vi "LSMcontroller_v62_updatedpointscan.vi"() -> ()   [LabVIEW 2015] (continued)
                                n918 = Transpose 2D Array(2D array=w3216) -> (transposed array=w3210:u16[][])
                                n919 = Transpose 2D Array(2D array=w3214) -> (transposed array=w3215:sgl[][])
                                n920 = And(x=w3220, y=w3209) -> (x .and. y?=w3222:bool)
                                n921 = local write "img_CH2"(w3215) -> ()
                                n922 = local write "photons/frame"(w3208) -> ()
                                n923 = Array Max & Min(array=w3210) -> (max value=w3211:u16)  [unwired: 3 out]
                                n924 = To Single Precision Float(number=w3210) -> (single precision float=w3213:sgl[][])
                                n925 = case shown="True" w3222 {
                                tunnel: w3221 -> [_ w3226]
                                frame False {
                                }
                                frame True {
                                n926 = Quotient & Remainder(x=w3226, y=u32 2 ("min phot")) -> (floor(x/y)=w3225:u32)  [unwired: 1 out]
                                n927 = Max & Min(x=w3225, y=u32 5) -> (max(x,y)=w3224:u32)  [unwired: 1 out]
                                n928 = local write "min phot"(w3224) -> ()
                                }
                                }
                                n929 = To Double Precision Float(number=w3211) -> (double precision float=w3212:dbl)
                                n930 = local write "img_CH1"(w3213) -> ()
                                n931 = property on="img_CH1" class="IntGraph (strict)"("ZScale.Maximum"=w3212) -> ()  [unwired: 2 in, 2 out]
                                }
                                }
                                }
                                frame #4 {
                                w3230 = u16 1 items=["Stream to disk", "Post process", "real time process"] ("Ring")
                                n932 = local read "T3R Data processing"() -> (w3229:u16)
                                n933 = Equal?(x=w3229, y=w3230) -> (x = y?=w3228:bool)
                                n934 = case shown="False" w3228 {
                                frame False {
                                # "intensity"
                                n935 = local read "Current Average"() -> (w3235:sgl)
                                n936 = local read "image2list"() -> (w3231:u16)
                                n937 = local read "image1list"() -> (w3232:u16)
                                n938 = call "dattoimage.vi"("image2list"=w3231, "Current Average"=w3235, "image1list"=w3232) -> ("image 1 array out"=w3234:sgl[][])  [unwired: 1 out]
                                n939 = Transpose 2D Array(2D array=w3234) -> (transposed array=w3233:sgl[][])
                                n940 = local write "img_CH2"(w3233) -> ()
                                }
                                frame True {
                                }
                                }
                                }
                                }
                              }
                              frame Enabled {
                              }
                            }
                          }
                        }
                        n941 = local write "64bit disabled"(TRUE ("64bit disabled")) -> ()
                      }
                      frame #9 {
                        n942 = call "2pparameters.vi"("command"="get") -> ("params out"=w3238:T10)  [unwired: 1 in]
                        n943 = Unbundle By Name(w3238) -> ("auto OD"=w3237:bool)
                        n944 = case shown="True" w3237 {
                          frame False {
                          }
                          frame True {
                            n945 = call "configuration.vi"("command"="get") -> ("config out"=w3241:T11)  [unwired: 2 in, 1 out]
                            n946 = call "2pparameters.vi"("command"="get") -> ("params out"=w3244:T10)  [unwired: 1 in]
                            n947 = Unbundle By Name(w3241) -> ("image OD"=w3239:u16)
                            n948 = Unbundle By Name(w3244) -> ("ODfilt"=w3240:u16)
                            n949 = call "filterwheelcontrol_nothorlabslib.vi"("Current OD filt"=w3239, "New ODfilt"=w3240) -> ()  [unwired: 1 in]
                          }
                        }
                        n950 = call "reset AO_DO_v3.vi"() -> ()  [unwired: 12 in]
                      }
                      frame #10 {
                        n951 = stacked-sequence {
                          tunnel: w3258 -> [w3261 _ _ _ _ _]
                          tunnel: w3257 -> [w3260 _ _ _ _ _]
                          tunnel: w3256 -> [w3259 _ _ _ _ _]
                          tunnel: w3255 -> [_ w3310 _ _ _ _]
                          tunnel: w3254 -> [_ w3309 w3364 w3461 _ _]
                          tunnel: w3253 -> [_ w3308 w3363 w3460 _ _]
                          tunnel: w3252 -> [_ _ w3362 _ _ _]
                          tunnel: w3251 -> [_ _ w3361 _ _ _]
                          tunnel: w3250 -> [_ _ _ w3459 _ _]
                          tunnel: w3249 -> [_ _ _ w3458 _ _]
                          tunnel: w3248 -> [_ _ w3359 _ _ _]
                          tunnel: w3247 -> [_ _ w3358 _ _ _]
                          tunnel: w3246 -> [_ _ _ w3456 _ _]
                          tunnel: w3245 -> [_ _ _ w3455 _ _]
                          frame #0 {
                            n952 = case shown="False" w3261 {
                              tunnel: w3260 -> [_ w3283]
                              tunnel: w3259 -> [_ w3282]
                              frame True {
                                n953 = stacked-sequence {
                                seq-local: [w3262 _ _] -> [_ w3274 w3279]
                                frame #0 {
                                n954 = call "configuration.vi"("command"="get") -> ("config out"=w3268:T11)  [unwired: 2 in, 1 out]
                                n955 = Unbundle By Name(w3268) -> ("Voltage to Xgalvo"=w3265:i32)
                                n956 = call "2pparameters.vi"("command"="get") -> ("params out"=w3266:T10)  [unwired: 1 in]
                                n957 = in-place {
                                in-place-border: w3265 -> [w3273]
                                in-place-border: [w3270] -> w3262
                                n958 = in-place-cluster #9(w3266) -> ("aAO"=w3272:u32[])
                                n959 = call "remove channel from active arrayv2.vi"("line array in"=w3272, "line to remove"=w3273) -> ("line array out"=w3271:u32[], "index"=w3270:i32)  [unwired: 1 out]
                                n960 = in-place-cluster #9("aAO"=w3271) -> (w3263:T10)
                                }
                                n961 = call "2pparameters.vi"("Params in"=w3263, "command"="set") -> ()  [unwired: 1 out]
                                }
                                frame #1 {
                                n962 = call "waveformparamsv2.vi"("command"="rem AO", "index"=w3274) -> ()  [unwired: 3 in, 3 out]
                                }
                                frame #2 {
                                n963 = call "waveformsAObuffer.vi"("command"="get") -> ("AO wf out"=w3280:waveform(dbl)[])  [unwired: 1 in]
                                n964 = Delete From Array(array=w3280, length=1, index=w3279) -> (array with subset deleted=w3276:waveform(dbl)[])  [unwired: 1 out]
                                n965 = call "waveformsAObuffer.vi"("AO wf in"=w3276, "command"="set") -> ()  [unwired: 1 out]
                                }
                                }
                              }
                              frame False {
                                n966 = stacked-sequence {
                                seq-local: [w3284 _ _] -> [_ w3292 w3303]
                                tunnel: w3283 -> [_ w3291 _]
                                tunnel: w3282 -> [_ _ w3302]
                                frame #0 {
                                n967 = call "configuration.vi"("command"="get") -> ("config out"=w3289:T11)  [unwired: 2 in, 1 out]
                                n968 = Unbundle By Name(w3289) -> ("Voltage to Xgalvo"=w3285:i32)
                                n969 = call "2pparameters.vi"("command"="get") -> ("params out"=w3288:T10)  [unwired: 1 in]
                                n970 = Unbundle By Name(w3288) -> ("aAO"=w3286:u32[])
                                n971 = Search 1D Array(1D array=w3286, element=w3285) -> (index of element=w3284:i32)  [unwired: 1 in]
                                }
                                frame #1 {
                                n972 = call "waveformparamsv2.vi"("command"="get") -> ("Params out"=w3295:T14)  [unwired: 4 in, 2 out]
                                n973 = in-place {
                                in-place-border: w3292 -> [w3299]
                                in-place-border: w3291 -> [w3298]
                                n974 = in-place-cluster #10(w3295) -> ("AO parameters"=w3300:T15)
                                n975 = in-place {
                                in-place-border: w3298 -> [w3301]
                                n976 = in-place-array #11(w3300, w3299) -> ()  [unwired: 1 out]
                                n977 = in-place-array #11(w3301) -> (w3297:T15)  [unwired: 1 out]
                                }
                                n978 = in-place-cluster #10("AO parameters"=w3297) -> (w3293:T14)
                                }
                                n979 = call "waveformparamsv2.vi"("command"="set", "Params in"=w3293) -> ()  [unwired: 3 in, 3 out]
                                }
                                frame #2 {
                                n980 = call "waveformsAObuffer.vi"("command"="get") -> ("AO wf out"=w3306:waveform(dbl)[])  [unwired: 1 in]
                                n981 = Replace Array Subset(array=w3306, new element=w3302, index=w3303) -> (w3304:waveform(dbl)[])
                                n982 = call "waveformsAObuffer.vi"("AO wf in"=w3304, "command"="set") -> ()  [unwired: 1 out]
                                }
                                }
                              }
                            }
                          }
                          frame #1 {
                            n983 = case shown="True" w3310 {
                              tunnel: w3309 -> [_ w3332]
                              tunnel: w3308 -> [_ w3331]
                              frame True {
                                n984 = stacked-sequence {
                                seq-local: [w3311 _ _] -> [_ w3323 w3328]
                                frame #0 {
                                n985 = call "configuration.vi"("command"="get") -> ("config out"=w3317:T11)  [unwired: 2 in, 1 out]
                                n986 = Unbundle By Name(w3317) -> ("Voltage to Ygalvo"=w3314:i32)
                                n987 = call "2pparameters.vi"("command"="get") -> ("params out"=w3315:T10)  [unwired: 1 in]
                                n988 = in-place {
                                in-place-border: w3314 -> [w3322]
                                in-place-border: [w3319] -> w3311
                                n989 = in-place-cluster #12(w3315) -> ("aAO"=w3321:u32[])
                                n990 = call "remove channel from active arrayv2.vi"("line array in"=w3321, "line to remove"=w3322) -> ("line array out"=w3320:u32[], "index"=w3319:i32)  [unwired: 1 out]
                                n991 = in-place-cluster #12("aAO"=w3320) -> (w3312:T10)
                                }
                                n992 = call "2pparameters.vi"("Params in"=w3312, "command"="set") -> ()  [unwired: 1 out]
                                }
                                frame #1 {
                                n993 = call "waveformparamsv2.vi"("command"="rem AO", "index"=w3323) -> ()  [unwired: 3 in, 3 out]
                                }
                                frame #2 {
                                n994 = call "waveformsAObuffer.vi"("command"="get") -> ("AO wf out"=w3329:waveform(dbl)[])  [unwired: 1 in]
                                n995 = Delete From Array(array=w3329, length=1, index=w3328) -> (array with subset deleted=w3325:waveform(dbl)[])  [unwired: 1 out]
                                n996 = call "waveformsAObuffer.vi"("AO wf in"=w3325, "command"="set") -> ()  [unwired: 1 out]
                                }
                                }
                              }
                              frame False {
                                n997 = stacked-sequence {
                                seq-local: [w3333 _ _] -> [_ w3341 w3352]
                                tunnel: w3332 -> [_ w3340 _]
                                tunnel: w3331 -> [_ _ w3351]
                                frame #0 {
                                n998 = call "configuration.vi"("command"="get") -> ("config out"=w3338:T11)  [unwired: 2 in, 1 out]
                                n999 = Unbundle By Name(w3338) -> ("Voltage to Ygalvo"=w3334:i32)
                                n1000 = call "2pparameters.vi"("command"="get") -> ("params out"=w3337:T10)  [unwired: 1 in]
                                n1001 = Unbundle By Name(w3337) -> ("aAO"=w3335:u32[])
                                n1002 = Search 1D Array(1D array=w3335, element=w3334) -> (index of element=w3333:i32)  [unwired: 1 in]
                                }
                                frame #1 {
                                n1003 = call "waveformparamsv2.vi"("command"="get") -> ("Params out"=w3344:T14)  [unwired: 4 in, 2 out]
                                n1004 = in-place {
                                in-place-border: w3341 -> [w3348]
                                in-place-border: w3340 -> [w3347]
                                n1005 = in-place-cluster #13(w3344) -> ("AO parameters"=w3349:T15)
                                n1006 = in-place {
                                in-place-border: w3347 -> [w3350]
                                n1007 = in-place-array #14(w3349, w3348) -> ()  [unwired: 1 out]
                                n1008 = in-place-array #14(w3350) -> (w3346:T15)  [unwired: 1 out]
                                }
                                n1009 = in-place-cluster #13("AO parameters"=w3346) -> (w3342:T14)
                                }
                                n1010 = call "waveformparamsv2.vi"("command"="set", "Params in"=w3342) -> ()  [unwired: 3 in, 3 out]
                                }
                                frame #2 {
                                n1011 = call "waveformsAObuffer.vi"("command"="get") -> ("AO wf out"=w3355:waveform(dbl)[])  [unwired: 1 in]
                                n1012 = Replace Array Subset(array=w3355, new element=w3351, index=w3352) -> (w3353:waveform(dbl)[])
                                n1013 = call "waveformsAObuffer.vi"("AO wf in"=w3353, "command"="set") -> ()  [unwired: 1 out]
                                }
                                }
                              }
                            }
                          }
                          frame #2 {
                            n1014 = Build Array(w3359, w3358) -> (w3357:bool[])
                            n1015 = Boolean Array To Number(Boolean array=w3357) -> (number=w3360:u32)
                            n1016 = case shown="0" w3360 {
                              tunnel: w3364 -> [_ _ w3407]
                              tunnel: w3363 -> [_ _ w3406]
                              tunnel: w3362 -> [_ w3386 w3404]
                              tunnel: w3361 -> [_ w3385 w3405]
                              frame 1, Default {
                                n1017 = stacked-sequence {
                                seq-local: [w3365 _ _] -> [_ w3377 w3382]
                                frame #0 {
                                n1018 = call "configuration.vi"("command"="get") -> ("config out"=w3371:T11)  [unwired: 2 in, 1 out]
                                n1019 = Unbundle By Name(w3371) -> ("2P shutter"=w3368:i32)
                                n1020 = call "2pparameters.vi"("command"="get") -> ("params out"=w3369:T10)  [unwired: 1 in]
                                n1021 = in-place {
                                in-place-border: w3368 -> [w3376]
                                in-place-border: [w3373] -> w3365
                                n1022 = in-place-cluster #15(w3369) -> ("aDO"=w3375:u32[])
                                n1023 = call "remove channel from active arrayv2.vi"("line array in"=w3375, "line to remove"=w3376) -> ("line array out"=w3374:u32[], "index"=w3373:i32)  [unwired: 1 out]
                                n1024 = in-place-cluster #15("aDO"=w3374) -> (w3366:T10)
                                }
                                n1025 = call "2pparameters.vi"("Params in"=w3366, "command"="set") -> ()  [unwired: 1 out]
                                }
                                frame #1 {
                                n1026 = call "waveformparamsv2.vi"("command"="rem DO", "index"=w3377) -> ()  [unwired: 3 in, 3 out]
                                }
                                frame #2 {
                                n1027 = call "waveformsDObuffer.vi"("command"="get") -> ("DO wf out"=w3383:digitalwaveform[])  [unwired: 1 in]
                                n1028 = Delete From Array(array=w3383, length=1, index=w3382) -> (array with subset deleted=w3379:digitalwaveform[])  [unwired: 1 out]
                                n1029 = call "waveformsDObuffer.vi"("DO wf in"=w3379, "command"="set") -> ()  [unwired: 1 out]
                                }
                                }
                              }
                              frame 2 {
                                n1030 = stacked-sequence {
                                tunnel: w3386 -> [_ w3397 _]
                                tunnel: w3385 -> [_ _ w3401]
                                frame #0 {
                                n1031 = call "configuration.vi"("command"="get") -> ("config out"=w3388:T11)  [unwired: 2 in, 1 out]
                                n1032 = call "2pparameters.vi"("command"="get") -> ("params out"=w3392:T10)  [unwired: 1 in]
                                n1033 = Unbundle By Name(w3388) -> ("2P shutter"=w3387:i32)
                                n1034 = in-place {
                                in-place-border: w3387 -> [w3396]
                                n1035 = in-place-cluster #16(w3392) -> ("aDO"=w3395:u32[])
                                n1036 = call "add channel to active arrayv2.vi"("line array in"=w3395, "line to add"=w3396) -> ("line array out"=w3394:u32[])  [unwired: 2 out]
                                n1037 = in-place-cluster #16("aDO"=w3394) -> (w3390:T10)
                                }
                                n1038 = call "2pparameters.vi"("Params in"=w3390, "command"="set") -> ()  [unwired: 1 out]
                                }
                                frame #1 {
                                n1039 = call "waveformparamsv2.vi"("command"="add DO", "add DO"=w3397) -> ()  [unwired: 3 in, 3 out]
                                }
                                frame #2 {
                                n1040 = call "waveformsDObuffer.vi"("command"="get") -> ("DO wf out"=w3402:digitalwaveform[])  [unwired: 1 in]
                                n1041 = Build Array (concatenate)(w3402, w3401) -> (w3400:digitalwaveform[])
                                n1042 = call "waveformsDObuffer.vi"("DO wf in"=w3400, "command"="set") -> ()  [unwired: 1 out]
                                }
                                }
                              }
                              frame 0 {
                                n1043 = stacked-sequence {
                                seq-local: [w3408 _ _] -> [_ w3416 w3438]
                                tunnel: w3407 -> [_ _ _]
                                tunnel: w3406 -> [_ _ _]
                                tunnel: w3405 -> [_ _ w3437]
                                tunnel: w3404 -> [_ w3415 _]
                                frame #0 {
                                n1044 = call "configuration.vi"("command"="get") -> ("config out"=w3413:T11)  [unwired: 2 in, 1 out]
                                n1045 = call "2pparameters.vi"("command"="get") -> ("params out"=w3412:T10)  [unwired: 1 in]
                                n1046 = Unbundle By Name(w3413) -> ("2P shutter"=w3409:i32)
                                n1047 = Unbundle By Name(w3412) -> ("aDO"=w3410:u32[])
                                n1048 = Search 1D Array(1D array=w3410, element=w3409) -> (index of element=w3408:i32)  [unwired: 1 in]
                                }
                                frame #1 {
                                n1049 = call "2pparameters.vi"("command"="get") -> ("params out"=w3419:T10)  [unwired: 1 in]
                                n1050 = Unbundle By Name(w3419) -> ("wavdet"=w3417:bool, "autoshutter"=w3418:bool)
                                n1051 = case shown="True" w3418 {
                                tunnel: w3416 -> [_ w3423]
                                tunnel: w3417 -> [_ w3422]
                                tunnel: w3415 -> [_ w3421]
                                frame False {
                                }
                                frame True {
                                n1052 = case shown="False" w3422 {
                                tunnel: w3423 -> [w3427 _]
                                tunnel: w3421 -> [w3425 _]
                                frame False {
                                n1053 = Index Array(array=w3425, index=0) -> (element=w3424:T18)
                                n1054 = call "waveformparamsv2.vi"("command"="get") -> ("Params out"=w3430:T14)  [unwired: 4 in, 2 out]
                                n1055 = in-place {
                                in-place-border: w3427 -> [w3434]
                                in-place-border: w3424 -> [w3432]
                                n1056 = in-place-cluster #17(w3430) -> ("DO parameters"=w3435:T17)
                                n1057 = in-place {
                                in-place-border: w3432 -> [w3436]
                                n1058 = in-place-array #18(w3435, w3434) -> ()  [unwired: 1 out]
                                n1059 = in-place-array #18(w3436) -> (w3433:T17)  [unwired: 1 out]
                                }
                                n1060 = in-place-cluster #17("DO parameters"=w3433) -> (w3428:T14)
                                }
                                n1061 = call "waveformparamsv2.vi"("command"="set", "Params in"=w3428) -> ()  [unwired: 3 in, 3 out]
                                }
                                frame True {
                                }
                                }
                                }
                                }
                                }
                                frame #2 {
                                n1062 = call "2pparameters.vi"("command"="get") -> ("params out"=w3441:T10)  [unwired: 1 in]
                                n1063 = Unbundle By Name(w3441) -> ("wavdet"=w3439:bool, "autoshutter"=w3440:bool)
                                n1064 = case shown="True" w3440 {
                                tunnel: w3438 -> [_ w3445]
                                tunnel: w3439 -> [_ w3444]
                                tunnel: w3437 -> [_ w3443]
                                frame False {
                                }
                                frame True {
                                n1065 = case shown="False" w3444 {
                                tunnel: w3445 -> [w3449 _]
                                tunnel: w3443 -> [w3448 _]
                                frame False {
                                n1066 = Index Array(array=w3448, index=0) -> (element=w3446:digitalwaveform)
                                n1067 = call "waveformsDObuffer.vi"("command"="get") -> ("DO wf out"=w3451:digitalwaveform[])  [unwired: 1 in]
                                n1068 = Replace Array Subset(array=w3451, new element=w3446, index=w3449) -> (w3453:digitalwaveform[])
                                n1069 = call "waveformsDObuffer.vi"("DO wf in"=w3453, "command"="set") -> ()  [unwired: 1 out]
                                }
                                frame True {
                                }
                                }
                                }
                                }
                                }
                                }
                              }
                            }
                          }
                          frame #3 {
                            n1070 = Build Array(w3456, w3455) -> (w3457:bool[])
                            n1071 = Boolean Array To Number(Boolean array=w3457) -> (number=w3454:u32)
                            n1072 = case shown="0" w3454 {
                              tunnel: w3461 -> [_ _ w3504]
                              tunnel: w3460 -> [_ _ w3503]
                              tunnel: w3459 -> [_ w3483 w3501]
                              tunnel: w3458 -> [_ w3482 w3502]
                              frame 1, Default {
                                n1073 = stacked-sequence {
                                seq-local: [w3462 _ _] -> [_ w3474 w3479]
                                frame #0 {
                                n1074 = call "configuration.vi"("command"="get") -> ("config out"=w3468:T11)  [unwired: 2 in, 1 out]
                                n1075 = Unbundle By Name(w3468) -> ("LT timestamp"=w3465:u32)
                                n1076 = call "2pparameters.vi"("command"="get") -> ("params out"=w3466:T10)  [unwired: 1 in]
                                n1077 = in-place {
                                in-place-border: w3465 -> [w3473]
                                in-place-border: [w3470] -> w3462
                                n1078 = in-place-cluster #19(w3466) -> ("aDO"=w3472:u32[])
                                n1079 = call "remove channel from active arrayv2.vi"("line array in"=w3472, "line to remove"=w3473) -> ("line array out"=w3471:u32[], "index"=w3470:i32)  [unwired: 1 out]
                                n1080 = in-place-cluster #19("aDO"=w3471) -> (w3463:T10)
                                }
                                n1081 = call "2pparameters.vi"("Params in"=w3463, "command"="set") -> ()  [unwired: 1 out]
                                }
                                frame #1 {
                                n1082 = call "waveformparamsv2.vi"("command"="rem DO", "index"=w3474) -> ()  [unwired: 3 in, 3 out]
                                }
                                frame #2 {
                                n1083 = call "waveformsDObuffer.vi"("command"="get") -> ("DO wf out"=w3480:digitalwaveform[])  [unwired: 1 in]
                                n1084 = Delete From Array(array=w3480, length=1, index=w3479) -> (array with subset deleted=w3476:digitalwaveform[])  [unwired: 1 out]
                                n1085 = call "waveformsDObuffer.vi"("DO wf in"=w3476, "command"="set") -> ()  [unwired: 1 out]
                                }
                                }
                              }
                              frame 2 {
                                n1086 = stacked-sequence {
                                tunnel: w3483 -> [_ _ w3496]
                                tunnel: w3482 -> [_ w3494 _]
                                frame #0 {
                                n1087 = call "configuration.vi"("command"="get") -> ("config out"=w3485:T11)  [unwired: 2 in, 1 out]
                                n1088 = Unbundle By Name(w3485) -> ("LT timestamp"=w3484:u32)
                                n1089 = call "2pparameters.vi"("command"="get") -> ("params out"=w3489:T10)  [unwired: 1 in]
                                n1090 = in-place {
                                in-place-border: w3484 -> [w3493]
                                n1091 = in-place-cluster #20(w3489) -> ("aDO"=w3492:u32[])
                                n1092 = call "add channel to active arrayv2.vi"("line array in"=w3492, "line to add"=w3493) -> ("line array out"=w3491:u32[])  [unwired: 2 out]
                                n1093 = in-place-cluster #20("aDO"=w3491) -> (w3487:T10)
                                }
                                n1094 = call "2pparameters.vi"("Params in"=w3487, "command"="set") -> ()  [unwired: 1 out]
                                }
                                frame #1 {
                                n1095 = call "waveformparamsv2.vi"("command"="add DO", "add DO"=w3494) -> ()  [unwired: 3 in, 3 out]
                                }
                                frame #2 {
                                n1096 = call "waveformsDObuffer.vi"("command"="get") -> ("DO wf out"=w3499:digitalwaveform[])  [unwired: 1 in]
                                n1097 = Build Array (concatenate)(w3499, w3496) -> (w3498:digitalwaveform[])
                                n1098 = call "waveformsDObuffer.vi"("DO wf in"=w3498, "command"="set") -> ()  [unwired: 1 out]
                                }
                                }
                              }
                              frame 0 {
                                n1099 = stacked-sequence {
                                seq-local: [w3505 _ _] -> [_ w3515 w3532]
                                tunnel: w3504 -> [_ _ _]
                                tunnel: w3503 -> [_ _ _]
                                tunnel: w3502 -> [_ w3512 _]
                                tunnel: w3501 -> [_ _ w3531]
                                frame #0 {
                                n1100 = call "configuration.vi"("command"="get") -> ("config out"=w3510:T11)  [unwired: 2 in, 1 out]
                                n1101 = Unbundle By Name(w3510) -> ("LT timestamp"=w3506:u32)
                                n1102 = call "2pparameters.vi"("command"="get") -> ("params out"=w3509:T10)  [unwired: 1 in]
                                n1103 = Unbundle By Name(w3509) -> ("aDO"=w3507:u32[])
                                n1104 = Search 1D Array(1D array=w3507, element=w3506) -> (index of element=w3505:i32)  [unwired: 1 in]
                                }
                                frame #1 {
                                n1105 = local read "Measurement"() -> (w3514:T4)
                                n1106 = To Unsigned Long Integer(number=w3514) -> (unsigned 32bit integer=w3513:u32)
                                n1107 = case shown="5..7" w3513 {
                                tunnel: w3515 -> [_ w3519]
                                tunnel: w3512 -> [_ w3516]
                                frame 0..4, Default {
                                }
                                frame 5..7 {
                                n1108 = Index Array(array=w3516, index=0) -> (element=w3517:T18)
                                n1109 = call "waveformparamsv2.vi"("command"="get") -> ("Params out"=w3522:T14)  [unwired: 4 in, 2 out]
                                n1110 = in-place {
                                in-place-border: w3519 -> [w3526]
                                in-place-border: w3517 -> [w3524]
                                n1111 = in-place-cluster #21(w3522) -> ("DO parameters"=w3527:T17)
                                n1112 = in-place {
                                in-place-border: w3524 -> [w3528]
                                n1113 = in-place-array #22(w3527, w3526) -> ()  [unwired: 1 out]
                                n1114 = in-place-array #22(w3528) -> (w3525:T17)  [unwired: 1 out]
                                }
                                n1115 = in-place-cluster #21("DO parameters"=w3525) -> (w3520:T14)
                                }
                                n1116 = call "waveformparamsv2.vi"("command"="set", "Params in"=w3520) -> ()  [unwired: 3 in, 3 out]
                                }
                                }
                                }
                                frame #2 {
                                n1117 = local read "Measurement"() -> (w3530:T4)
                                n1118 = To Unsigned Long Integer(number=w3530) -> (unsigned 32bit integer=w3529:u32)
                                n1119 = case shown="5..7" w3529 {
                                tunnel: w3532 -> [_ w3536]
                                tunnel: w3531 -> [_ w3534]
                                frame 0..4, Default {
                                }
                                frame 5..7 {
                                n1120 = Index Array(array=w3534, index=0) -> (element=w3533:digitalwaveform)
                                n1121 = call "waveformsDObuffer.vi"("command"="get") -> ("DO wf out"=w3538:digitalwaveform[])  [unwired: 1 in]
                                n1122 = Replace Array Subset(array=w3538, new element=w3533, index=w3536) -> (w3540:digitalwaveform[])
                                n1123 = call "waveformsDObuffer.vi"("DO wf in"=w3540, "command"="set") -> ()  [unwired: 1 out]
                                }
                                }
                                }
                                }
                              }
                            }
                          }
                          frame #4 {
                            n1124 = call "Used AO lines.vi"() -> ("used AO names"=w3543:string[], "used AO lines"=w3541:tag[])  [unwired: 2 in]
                            n1125 = control-ref of="Analog Lines Plot"() -> (w3542:refnum<vi>)
                            n1126 = control-ref of="Digital Lines Plot"() -> (w3544:refnum<vi>)
                            n1127 = call "Used DO lines.vi"() -> ("used DO names"=w3545:string[], "used DO lines"=w3546:tag[])  [unwired: 2 in]
                            n1128 = local write "Analog Used Lines"(w3541) -> ()
                            n1129 = local write "Analog Used Names"(w3543) -> ()
                            n1130 = local write "Digital Used Lines"(w3546) -> ()
                            n1131 = local write "Digital Used Names"(w3545) -> ()
                            n1132 = call "prepDOWaveplot.vi"("DigitalGraph in"=w3544, "used DO names"=w3545) -> ()  [unwired: 1 in]
                            n1133 = call "prepAOWaveplot.vi"("WaveformGraph in"=w3542, "Analog Used Names"=w3543) -> ()  [unwired: 1 in]
                          }
                          frame #5 {
                            n1134 = local read "Meastab"() -> (w3561:enum32{"X-Y Image", "Linescan", "Timetrace"})
                            n1135 = property on="refwf" class="Ring (strict)"() -> ("RingText.Text"=w3558:string)  [unwired: 2 in, 2 out]
                            n1136 = case shown="\"Timetrace\"" w3561 {
                              tunnel: [w3563 w3564] -> w3562
                              frame "X-Y Image", Default {
                                n1137 = local read "Sampling rate"() -> (w3563:dbl)
                              }
                              frame "Timetrace" {
                                n1138 = local read "srateAODOtt"() -> (w3564:dbl)
                              }
                            }
                            n1139 = call "waveformsAObuffer.vi"("command"="get") -> ("AO wf out"=w3549:waveform(dbl)[])  [unwired: 1 in]
                            n1140 = local read "wavdet"() -> (w3559:bool)
                            n1141 = call "waveformsDObuffer.vi"("command"="get") -> ("DO wf out"=w3553:digitalwaveform[])  [unwired: 1 in]
                            n1142 = call "correctwaveformsizetemp.vi"("new sampling frequency (Hz)"=w3562, "start"=FALSE, "reference waveforms to"=w3558, "Analog waveforms in"=w3549, "stop"=TRUE, "Digital waveforms in"=w3553) -> ("analog wf out"=w3555:waveform(dbl)[], "Digital wf out"=w3557:digitalwaveform[], "measpoints"=w3560:i32)
                            n1143 = local write "Analog Lines Plot"(w3555) -> ()
                            n1144 = call "GetNumCamFramesv2.vi"("Digital Waveform Graph"=w3557) -> ("Numeric"=w3556:i32)  [unwired: 10 in]
                            n1145 = local write "Digital Lines Plot"(w3557) -> ()
                            n1146 = call "waveformsDObuffer.vi"("DO wf in"=w3557, "command"="set") -> ()  [unwired: 1 out]
                            n1147 = call "waveformsAObuffer.vi"("AO wf in"=w3555, "command"="set") -> ()  [unwired: 1 out]
                            n1148 = local write "Total Camera Frames"(w3556) -> ()
                            n1149 = case shown="True" w3559 {
                              tunnel: w3560 -> [_ w3565]
                              frame False {
                              }
                              frame True {
                                n1150 = local write "# of frames"(w3565) -> ()
                              }
                            }
                          }
                        }
                        n1151 = call "stoperaseCI.vi"() -> ()  [unwired: 12 in]
                        n1152 = call "stoperaseDO_img.vi"() -> ()  [unwired: 12 in]
                        n1153 = call "stoperaseAO_img.vi"() -> ()  [unwired: 12 in]
                        n1154 = call "stoperaseAI_img.vi"() -> ()  [unwired: 12 in]
                      }
                      frame #11 {
                        w3573 = FALSE ("Value (Signaling)")
                        n1155 = local read "save\ndata"() -> (w3566:bool)
                        n1156 = local read "save\ndata"() -> (w3567:bool)
                        n1157 = property on="Stop" class="Bool (strict)"("Visible"=FALSE, "DisabledEnum"=T7."Disabled" ("Disabled")) -> ()  [unwired: 2 in, 2 out]
                        n1158 = case shown="True" w3566 {
                          frame False {
                          }
                          frame True {
                            n1159 = call "closetiffs.vi"() -> ()  [unwired: 12 in]
                          }
                        }
                        n1160 = case shown="True" w3567 {
                          tunnel: w3568 -> [_ w3574]
                          frame False {
                          }
                          frame True {
                            n1161 = local read "filename prefix"() -> (w3576:string)
                            n1162 = local read "data dir"() -> (w3575:path)
                            n1163 = call "savetimestamps.vi"("timestamp"=w3574, "filename prefix in"=w3576, "data dir in"=w3575) -> ()  [unwired: 1 in]
                            n1164 = call "saveparams.vi"("filename prefix in"=w3576, "data dir in"=w3575) -> ()  [unwired: 2 in]
                          }
                        }
                        n1165 = property on="Start" class="Bool (strict)"("Visible"=TRUE, "DisabledEnum"=T7."Enabled" ("Disabled")) -> ()  [unwired: 2 in, 2 out]
                        n1166 = property on="Start" class="Bool (strict)"("Val(Sgnl)"=w3573) -> ()  [unwired: 2 in, 2 out]
                        n1167 = property on="Stop" class="Bool (strict)"("Val(Sgnl)"=w3573) -> ()  [unwired: 2 in, 2 out]
                      }
                      frame #12 {
                        w3580 = T21 2 items=["no dialog", "OK message", "continue or stop message", "OK message + warnings", "continue/stop + warnings"] ("type of dialog (OK msg:1)")
                        n1168 = call "displayerrors.vi"() -> ("error IO"=w3579:errorcluster)
                        n1169 = call <vilib>:"General Error Handler.vi"("type of dialog (OK msg:1)"=w3580, "error in (no error)"=w3579) -> ("error out"=w3578:errorcluster)  [unwired: 9 in, 4 out]
                        n1170 = call <vilib>:"Clear Errors.vi"("error in (no error)"=w3578) -> ("error out"=w3577:errorcluster)  [unwired: 5 in, 1 out]
                        n1171 = call "seterrors.vi"("error IO"=w3577) -> ()
                      }
                    }
                  }
                  frame "X-Y-Z-t movie" {
                    n1172 = call "2pparameters.vi"("command"="get") -> ("params out"=w3583:T10)  [unwired: 1 in]
                    n1173 = Bundle By Name(cluster=w3583, "type"="X-Y-Z-t movie") -> (w3581:T10)
                    n1174 = call "2pparameters.vi"("Params in"=w3581, "command"="set") -> ()  [unwired: 1 out]
                  }
                  frame "linescan" {
                    n1175 = call "2pparameters.vi"("command"="get") -> ("params out"=w3588:T10)  [unwired: 1 in]
                    n1176 = Bundle By Name(cluster=w3588, "type"="linescan") -> (w3590:T10)
                    n1177 = call "2pparameters.vi"("Params in"=w3590, "command"="set") -> ()  [unwired: 1 out]
                  }
                  frame "Timetrace", "Lifetime (contour)" {
                    n1178 = local read "ttt"() -> (w3591:T3)
                    n1179 = case shown="\"Point\", \"Resonant Ellipse\", \"freeform contour\", \"Fill Ellipse\", Default" w3591 {
                      selector: w3591 -> [_ w3592]
                      frame "Line" {
                      }
                      frame "Point", "Resonant Ellipse", "freeform contour", "Fill Ellipse", Default {
                        n1180 = stacked-sequence {
                          seq-local: [w3608 _ _ _ _ _ _ _ _ _ _] -> [_ _ w4481 _ _ w4494 w4561 _ _ w4921 _]
                          seq-local: [w3607 _ _ _ _ _ _ _ _ _ _] -> [_ _ _ _ _ _ _ _ w4608 _ _]
                          seq-local: [w3606 _ _ _ _ _ _ _ _ _ _] -> [_ _ _ _ _ _ _ _ w4607 _ _]
                          seq-local: [w3605 _ _ _ _ _ _ _ _ _ _] -> [_ _ _ _ _ _ _ _ w4610 _ _]
                          seq-local: [w3604 _ _ _ _ _ _ _ _ _ _] -> [_ _ _ _ _ _ _ _ w4606 _ _]
                          seq-local: [w3603 _ _ _ _ _ _ _ _ _ _] -> [_ _ _ _ _ _ _ _ w4605 _ _]
                          seq-local: [w3602 _ _ _ _ _ _ _ _ _ _] -> [_ _ _ _ _ _ _ _ w4609 _ _]
                          seq-local: [w3601 _ _ _ _ _ _ _ _ _ _] -> [_ _ _ _ _ _ _ _ w4604 _ _]
                          seq-local: [w3600 _ _ _ _ _ _ _ _ _ _] -> [_ _ _ _ _ _ _ _ w4603 _ _]
                          seq-local: [w3599 _ _ _ _ _ _ _ _ _ _] -> [_ _ _ _ _ _ _ _ w4598 _ _]
                          seq-local: [w3598 _ _ _ _ _ _ _ _ _ _] -> [_ _ _ _ _ _ _ _ w4597 _ _]
                          seq-local: [w3597 _ _ _ _ _ _ _ _ _ _] -> [_ _ _ _ _ _ _ _ w4602 _ _]
                          seq-local: [w3596 _ _ _ _ _ _ _ _ _ _] -> [_ _ _ _ _ _ _ _ w4601 _ _]
                          seq-local: [w3595 _ _ _ _ _ _ _ _ _ _] -> [_ _ _ _ _ _ _ _ w4600 _ _]
                          seq-local: [w3594 _ _ _ _ _ _ _ _ _ _] -> [_ _ _ _ _ _ _ _ w4599 _ _]
                          tunnel: w3592 -> [w3593 _ _ _ _ _ _ _ _ _ _]
                          frame #0 {
                            n1181 = local read "save\ndata"() -> (w3609:bool)
                            n1182 = Get Date/Time In Seconds() -> (seconds since 1Jan1904=w3610:timestamp)
                            n1183 = case shown="False" w3609 {
                              tunnel: w3610 -> [w3611 w3613]
                              tunnel: [w3611 w3612] -> w3608
                              frame False {
                              }
                              frame True {
                                n1184 = call "createdatafolder.vi"("timestamp in"=w3613) -> ("current data path"=w3614:path, "timestamp out"=w3612:timestamp)
                                n1185 = local write "data dir"(w3614) -> ()
                              }
                            }
                            n1186 = stacked-sequence {
                              tunnel: w3608 -> [w3620 _ _ _ _ _ _ _ _]
                              tunnel: [_ _ _ _ _ _ w3786 _ _] -> w3607
                              tunnel: [_ _ _ _ _ _ w3785 _ _] -> w3606
                              tunnel: [_ _ _ _ _ _ w3784 _ _] -> w3605
                              tunnel: [_ _ _ _ _ _ w3783 _ _] -> w3604
                              tunnel: [_ _ _ _ _ _ w3782 _ _] -> w3603
                              tunnel: [_ _ _ _ _ _ w3781 _ _] -> w3602
                              tunnel: [_ _ _ _ _ _ w3780 _ _] -> w3601
                              tunnel: [_ _ _ _ _ _ w3779 _ _] -> w3600
                              tunnel: [_ _ _ _ _ _ w3778 _ _] -> w3599
                              tunnel: [_ _ _ _ _ _ w3777 _ _] -> w3598
                              tunnel: [_ _ _ _ _ _ w3776 _ _] -> w3597
                              tunnel: [_ _ _ _ _ _ w3775 _ _] -> w3596
                              tunnel: [_ _ _ _ _ _ w3774 _ _] -> w3595
                              tunnel: [_ _ _ _ _ _ w3773 _ _] -> w3594
                              tunnel: w3593 -> [_ _ w3658 _ w3717 _ _ _ _]
                              frame #0 {
                                n1187 = local write "graphtab"(T5."timetrace" ("graphtab")) -> ()
                                n1188 = local read "AI channels"() -> (w3624:i32[])
                                n1189 = local read "CI channels"() -> (w3625:i32[])
                                n1190 = property on="Stop" class="Bool (strict)"("Visible"=TRUE, "DisabledEnum"=T7."Enabled" ("Disabled")) -> ()  [unwired: 2 in, 2 out]
                                n1191 = property on="Start" class="Bool (strict)"("Visible"=FALSE, "DisabledEnum"=T7."Disabled and Grayed Out" ("Disabled")) -> ()  [unwired: 2 in, 2 out]
                                n1192 = Format Date/Time String(time format string (%c)="%Y%m%d", seconds (now)=w3620) -> (date/time string=w3619:string)  [unwired: 1 in]
                                n1193 = Format Date/Time String(time format string (%c)="%H%M%S", seconds (now)=w3620) -> (date/time string=w3618:string)  [unwired: 1 in]
                                n1194 = call "2pparameters.vi"("command"="get") -> ("params out"=w3627:T10)  [unwired: 1 in]
                                n1195 = Bundle By Name(cluster=w3627, "aAI"=w3624, "aCI"=w3625, "type"="Timetrace", "date"=w3619, "time"=w3618) -> (w3626:T10)
                                n1196 = call "X-array-databuffer.vi"("command"=enum16{"get", "set", "clear", "append"}."clear") -> ()  [unwired: 3 in, 2 out]
                                n1197 = call "Y-array-databuffer.vi"("command"=enum16{"get", "set", "clear", "append"}."clear") -> ()  [unwired: 3 in, 2 out]
                                n1198 = call "2pparameters.vi"("Params in"=w3626, "command"="set") -> ()  [unwired: 1 out]
                                n1199 = call "CH1-1D-temp.vi"("command"=enum16{"get", "set", "clear", "append"}."clear") -> ()  [unwired: 3 in, 2 out]
                                n1200 = call "CH2-1D-temp.vi"("command"=enum16{"get", "set", "clear", "append"}."clear") -> ()  [unwired: 3 in, 2 out]
                                n1201 = call "allAI-temp.vi"("command"=enum16{"get", "set", "clear", "append"}."clear") -> ()  [unwired: 3 in, 2 out]
                              }
                              frame #1 {
                                n1202 = call "configuration.vi"("command"="get") -> ("config out"=w3644:T11)  [unwired: 2 in, 1 out]
                                n1203 = Unbundle By Name(w3644) -> ("CI names"=w3645:string[], "AI names"=w3646:string[])
                                n1204 = call "2pparameters.vi"("command"="get") -> ("params out"=w3640:T10)  [unwired: 1 in]
                                n1205 = Unbundle By Name(w3640) -> ("aCI"=w3641:i32[], "aAI"=w3642:i32[])
                                n1206 = for {
                                tunnel: w3641 -> [w3656] mode=indexing
                                tunnel: w3645 -> [w3657]
                                tunnel: [w3655] -> w3647 mode=indexing
                                n1207 = Index Array(array=w3657, index=w3656) -> (element=w3655:string)
                                }
                                n1208 = for {
                                tunnel: w3642 -> [w3653] mode=indexing
                                tunnel: w3646 -> [w3654]
                                tunnel: [w3652] -> w3648 mode=indexing
                                n1209 = Index Array(array=w3654, index=w3653) -> (element=w3652:string)
                                }
                                n1210 = Build Array (concatenate)(w3647, w3648) -> (w3638:string[])
                                n1211 = for {
                                tunnel: w3638 -> [w3650] mode=indexing
                                tunnel: [w3649] -> w3637 mode=indexing
                                i -> [w3651]
                                n1212 = Bundle("String"=w3650, w3651) -> (w3649:cluster{"String":string, i32})  [unwired: 1 in]
                                }
                                n1213 = property on="graph1list" class="Ring (strict)"("StringsAndValues[]"=w3637) -> ()  [unwired: 2 in, 2 out]
                                n1214 = property on="graph2list" class="Ring (strict)"("StringsAndValues[]"=w3637) -> ()  [unwired: 2 in, 2 out]
                              }
                              frame #2 {
                                n1215 = call "2pparameters.vi"("command"="get") -> ("params out"=w3661:T10)  [unwired: 1 in]
                                n1216 = Unbundle By Name(w3661) -> ("auto OD"=w3659:bool, "autoshutter"=w3662:bool)
                                n1217 = case shown="True" w3659 {
                                tunnel: w3658 -> [_ w3663]
                                frame False {
                                }
                                frame True {
                                n1218 = case shown="\"Point\"" w3663 {
                                frame "Point" {
                                n1219 = call "configuration.vi"("command"="get") -> ("config out"=w3666:T11)  [unwired: 2 in, 1 out]
                                n1220 = Unbundle By Name(w3666) -> ("point OD"=w3667:u16)
                                n1221 = local read "ODfilt"() -> (w3664:u16)
                                n1222 = call "filterwheelcontrol_nothorlabslib.vi"("Current OD filt"=w3664, "New ODfilt"=w3667) -> ()  [unwired: 1 in]
                                }
                                frame "Resonant Ellipse", Default {
                                n1223 = call "configuration.vi"("command"="get") -> ("config out"=w3670:T11)  [unwired: 2 in, 1 out]
                                n1224 = Unbundle By Name(w3670) -> ("contour OD"=w3671:u16)
                                n1225 = local read "ODfilt"() -> (w3668:u16)
                                n1226 = call "filterwheelcontrol_nothorlabslib.vi"("Current OD filt"=w3668, "New ODfilt"=w3671) -> ()  [unwired: 1 in]
                                }
                                }
                                }
                                }
                                n1227 = case shown="True" w3662 {
                                frame False {
                                }
                                frame True {
                                n1228 = call "shuttercontrol.vi"("command"="close") -> ()  [unwired: 1 in, 1 out]
                                }
                                }
                              }
                              frame #3 {
                                n1229 = local read "Vy-min draw"() -> (w3680:dbl)
                                n1230 = local read "Vy-max draw"() -> (w3679:dbl)
                                n1231 = local read "Vx-min draw"() -> (w3682:dbl)
                                n1232 = local read "Vx-max draw"() -> (w3681:dbl)
                                n1233 = local read "xpixels ref"() -> (w3678:i32)
                                n1234 = local read "ypixels ref"() -> (w3677:i32)
                                n1235 = local read "ROI Type"() -> (w3676:u16)
                                n1236 = local read "srateAODOtt"() -> (w3699:dbl)
                                n1237 = local read "# of frames"() -> (w3704:i32)
                                n1238 = local read "refreshtime"() -> (w3696:dbl)
                                n1239 = local read "Pel"() -> (w3675:dbl)
                                n1240 = local read "bin"() -> (w3702:dbl)
                                n1241 = local read "Override AI buffer"() -> (w3673:bool)
                                n1242 = local read "finite samples"() -> (w3711:bool)
                                n1243 = local read "srateAODOtt"() -> (w3698:dbl)
                                n1244 = local read "srateAODOtt"() -> (w3705:dbl)
                                n1245 = local read "continuous"() -> (w3710:bool)
                                n1246 = local read "Angle ref"() -> (w3683:dbl)
                                n1247 = local read "wavdet"() -> (w3712:bool)
                                n1248 = local read "Vx-ref"() -> (w3707:dbl)
                                n1249 = local read "Vy-ref"() -> (w3709:dbl)
                                n1250 = local read "avpp"() -> (w3708:i32)
                                n1251 = call "tt_timeandsamples.vi"("bin"=w3702, "refreshtime"=w3696, "srateAODOtt"=w3699, "tot#ofsamples"=w3704) -> ("refreshrate"=w3700:dbl, "refreshbuffer"=w3701:i32, "timetracecycles"=w3706:i32)  [unwired: 5 in]
                                n1252 = local read "bin"() -> (w3703:dbl)
                                n1253 = call "2pparameters.vi"("command"="get") -> ("params out"=w3715:T10)  [unwired: 1 in]
                                n1254 = Bundle By Name(cluster=w3715, "Drawing Mode"=w3676, "measpoints"=w3704, "tt_cycles"=w3706, "refreshbuffer"=w3701, "refreshrate"=w3700, "Vx-ref"=w3707, "Vy-ref"=w3709, "srate"=w3698, "finite"=w3711, "cont"=w3710, "wavdet"=w3712, "avpp"=w3708, "srateAODO"=w3705, "bufferAI"=w3701, "bin"=w3703, "Angle Img"=w3683, "Vxminref"=w3682, "Vxmaxref"=w3681, "Vyminref"=w3680, "Vymaxref"=w3679, "Xpixels Img"=w3678, "Ypixels Img"=w3677, "Pel"=w3675, "Vz-reset"=0.0, "AIoverride"=w3673) -> (w3713:T10)
                                n1255 = Reciprocal(x=w3700) -> (1/x=w3697:dbl)
                                n1256 = local write "refreshtime"(w3697) -> ()
                                n1257 = call "2pparameters.vi"("Params in"=w3713, "command"="set") -> ()  [unwired: 1 out]
                                n1258 = local read "Voltage Clamp"() -> (w3690:bool)
                                n1259 = local read "Current Clamp"() -> (w3691:bool)
                                n1260 = local read "Vholding (mV)"() -> (w3685:sgl)
                                n1261 = local read "CC_ICgain"() -> (w3689:dbl)
                                n1262 = local read "OCgain"() -> (w3686:sgl)
                                n1263 = local read "holdon"() -> (w3684:bool)
                                n1264 = call "patchparameters.vi"("command"="get") -> ("Params out"=w3693:T13)  [unwired: 1 in]
                                n1265 = Bundle By Name(cluster=w3693, "VC"=w3690, "CC"=w3691, "CC_icg (pA/mv)"=w3689, "VC_icg (mV/mV)"=10.0, "OCG (mV/pA)"=w3686, "OVG (mV/mV)"=0.1, "Vhold (mV)"=w3685, "holdon"=w3684) -> (w3692:T13)
                                n1266 = call "patchparameters.vi"("Params in"=w3692, "command"="set") -> ()  [unwired: 1 out]
                              }
                              frame #4 {
                                n1267 = case shown="\"Point\"" w3717 {
                                frame "Point" {
                                n1268 = call "2pparameters.vi"("command"="get") -> ("params out"=w3733:T10)  [unwired: 1 in]
                                n1269 = Unbundle By Name(w3733) -> ("Pel"=w3722:sgl, "Vx-min Img"=w3735:dbl, "VX-max Img"=w3734:dbl, "Vy-min Img"=w3737:dbl, "Vy-max Img"=w3736:dbl, "Angle Img"=w3738:dbl, "Vx-ref"=w3731:dbl, "Vy-ref"=w3730:dbl)
                                n1270 = script code="Xic=(ximax+ximin)./2;\nYic=(yimax+yimin)./2;\nx=x-Xic;\ny=y-Yic;\nxout=x.*cos(pi/180.*phi)+y.*sin(pi./180.*phi)+Xic;\nyout=-x.*sin(pi./180.*phi)+y.*cos(pi./180.*phi)+Yic;"("ximax"=w3734, "ximin"=w3735, "yimax"=w3736, "yimin"=w3737, "phi"=w3738, "x"=w3731, "y"=w3730) -> ("xout"=w3724:dbl, "yout"=w3723:dbl)  [unwired: 1 in, 1 out]
                                n1271 = call "2pparameters.vi"("command"="get") -> ("params out"=w3726:T10)  [unwired: 1 in]
                                n1272 = Bundle By Name(cluster=w3726, "P"=0.0) -> (w3729:T10)
                                n1273 = Initialize Array(w3723, w3722) -> (w3720:dbl[])
                                n1274 = Initialize Array(w3724, w3722) -> (w3719:dbl[])
                                n1275 = call "2pparameters.vi"("Params in"=w3729, "command"="set") -> ()  [unwired: 1 out]
                                n1276 = call "X-array-databuffer.vi"("array in"=w3719, "command"=enum16{"get", "set", "clear", "append"}."set") -> ()  [unwired: 2 in, 2 out]
                                n1277 = call "Y-array-databuffer.vi"("array in"=w3720, "command"=enum16{"get", "set", "clear", "append"}."set") -> ()  [unwired: 2 in, 2 out]
                                }
                                frame "Resonant Ellipse", Default {
                                n1278 = call "2pparameters.vi"("command"="get") -> ("params out"=w3753:T10)  [unwired: 1 in]
                                n1279 = Unbundle By Name(w3753) -> ("srateAODO"=w3754:sgl, "Angle Img"=w3755:dbl, "Angle draw"=w3756:dbl, "Vxmaxref"=w3757:dbl, "Vxminref"=w3758:dbl, "Xpixels Img"=w3759:i32, "Ypixels Img"=w3760:i32, "Vymaxref"=w3761:dbl, "Vxminref"=w3762:dbl, "Drawing Mode"=w3763:u16, "Pel"=w3764:sgl)
                                n1280 = Add(x=w3755, y=w3756) -> (x+y=w3739:dbl)
                                n1281 = call "ROI-databuffer.vi"("command"=enum16{"get", "set", "clear", "append"}."get") -> ("array out"=w3747:cluster{"x":sgl, "y":sgl}[])  [unwired: 4 in]
                                n1282 = call "ScanningWaveform_v4.vi"("Vy-min"=w3762, "Vy-max"=w3761, "yPixels/tPixels"=w3760, "xPixels/rPixels"=w3759, "Vx-min"=w3758, "Vx-max"=w3757, "Drawing Mode"=w3763, "Angle"=w3739, "AOrate"=w3754, "Points"=w3747, "points in ellipse"=w3764) -> ("numPixels"=w3740:dbl, "Y-WaveArray"=w3741:dbl[], "P"=w3746:dbl, "X-WaveArray"=w3742:dbl[])  [unwired: 5 in]
                                n1283 = call "Y-array-databuffer.vi"("array in"=w3741, "command"=enum16{"get", "set", "clear", "append"}."set") -> ()  [unwired: 2 in, 2 out]
                                n1284 = call "X-array-databuffer.vi"("array in"=w3742, "command"=enum16{"get", "set", "clear", "append"}."set") -> ()  [unwired: 2 in, 2 out]
                                n1285 = call "2pparameters.vi"("command"="get") -> ("params out"=w3751:T10)  [unwired: 1 in]
                                n1286 = Bundle By Name(cluster=w3751, "P"=w3746, "sAOxy"=w3740, "Pel"=w3740) -> (w3743:T10)
                                n1287 = call "2pparameters.vi"("Params in"=w3743, "command"="set") -> ()  [unwired: 1 out]
                                }
                                }
                              }
                              frame #5 {
                                n1288 = call "X-array-databuffer.vi"("command"=enum16{"get", "set", "clear", "append"}."get") -> ("array out"=w3767:dbl[])  [unwired: 3 in, 1 out]
                                n1289 = call "Y-array-databuffer.vi"("command"=enum16{"get", "set", "clear", "append"}."get") -> ("array out"=w3770:dbl[])  [unwired: 3 in, 1 out]
                                n1290 = Index Array(array=w3767, index=0) -> (element=w3766:dbl)
                                n1291 = Index Array(array=w3770, index=0) -> (element=w3765:dbl)
                                n1292 = call "setposition.vi"("Vy"=w3765, "Vx"=w3766) -> ()  [unwired: 1 in]
                              }
                              frame #6 {
                                # "rem2Ps"
                                # "A2Ps"
                                # "Al"
                                # "Rl"
                                n1293 = stacked-sequence {
                                seq-local: [w3791 _ _ _ _ _ _ _ _ _ _] -> [_ w3903 _ w3964 _ w4050 _ _ _ _ _]
                                seq-local: [w3792 _ _ _ _ _ _ _ _ _ _] -> [_ w3904 w3914 _ w4019 _ _ _ _ _ _]
                                seq-local: [_ _ w3913 _ _ _ _ _ _ _ _] -> [_ _ _ _ w4013 _ _ _ _ _ _]
                                seq-local: [_ _ _ w3963 _ _ _ _ _ _ _] -> [_ _ _ _ _ w4049 _ _ _ _ _]
                                seq-local: [w3788 _ _ _ _ _ _ _ _ _ _] -> [_ w3900 _ _ _ _ _ _ w4235 w4303 _]
                                seq-local: [w3787 _ _ _ _ _ _ _ _ _ _] -> [_ w3899 _ _ _ _ _ _ w4236 w4304 _]
                                seq-local: [w3794 _ _ _ _ _ _ _ _ _ _] -> [_ _ _ _ _ _ w4088 _ w4234 w4302 _]
                                seq-local: [w3790 _ _ _ _ _ _ _ _ _ _] -> [_ w3898 _ _ _ _ w4087 w4155 _ _ _]
                                seq-local: [w3789 _ _ _ _ _ _ _ _ _ _] -> [_ w3897 _ _ _ _ w4086 w4154 _ _ _]
                                seq-local: [w3793 _ _ _ _ _ _ _ _ _ _] -> [_ _ _ _ _ _ w4085 w4153 _ _ _]
                                tunnel: [_ _ w3912 _ _ _ _ _ _ _ _] -> w3785
                                tunnel: [_ _ w3911 _ _ _ _ _ _ _ _] -> w3786
                                tunnel: [w3792 _ _ _ _ _ _ _ _ _ _] -> w3784
                                tunnel: [w3791 _ _ _ _ _ _ _ _ _ _] -> w3781
                                tunnel: [_ _ _ w3962 _ _ _ _ _ _ _] -> w3782
                                tunnel: [_ _ _ w3961 _ _ _ _ _ _ _] -> w3783
                                tunnel: [w3790 _ _ _ _ _ _ _ _ _ _] -> w3776
                                tunnel: [w3789 _ _ _ _ _ _ _ _ _ _] -> w3775
                                tunnel: [_ _ _ _ _ _ w4084 _ _ _ _] -> w3774
                                tunnel: [_ _ _ _ _ _ _ w4152 _ _ _] -> w3773
                                tunnel: [w3788 _ _ _ _ _ _ _ _ _ _] -> w3777
                                tunnel: [w3787 _ _ _ _ _ _ _ _ _ _] -> w3778
                                tunnel: [_ _ _ _ _ _ _ _ w4233 _ _] -> w3779
                                tunnel: [_ _ _ _ _ _ _ _ _ w4301 _] -> w3780
                                frame #0 {
                                # "for a next version, give ome thought to\nthe possibilit of intermittently updating the\nwaveforms. it will have to be a calculation\nbased on speed of CPU and program on the one hand\nand length of measurement on the other. but then it should be possible, in principle, to \nupdate the waveform on the fly and that way cut up a longer measurement in smaller parts."
                                n1294 = stacked-sequence {
                                tunnel: [w3795 _ _ _] -> w3792
                                tunnel: [_ w3807 _ _] -> w3791
                                tunnel: [_ _ _ w3864] -> w3787
                                tunnel: [_ _ _ w3863] -> w3788
                                tunnel: [_ _ _ w3862] -> w3794
                                tunnel: [_ _ w3822 _] -> w3790
                                tunnel: [_ _ w3821 _] -> w3789
                                tunnel: [_ _ w3820 _] -> w3793
                                frame #0 {
                                n1295 = call "configuration.vi"("command"="get") -> ("config out"=w3797:T11)  [unwired: 2 in, 1 out]
                                n1296 = Unbundle By Name(w3797) -> ("Voltage to Xgalvo"=w3796:i32)
                                n1297 = call "2pparameters.vi"("command"="get") -> ("params out"=w3801:T10)  [unwired: 1 in]
                                n1298 = in-place {
                                in-place-border: w3796 -> [w3806]
                                in-place-border: [w3803] -> w3795
                                n1299 = in-place-cluster #23(w3801) -> ("aAO"=w3805:u32[])
                                n1300 = call "add channel to active arrayv2.vi"("line array in"=w3805, "line to add"=w3806) -> ("line array out"=w3804:u32[], "addition"=w3803:bool)  [unwired: 1 out]
                                n1301 = in-place-cluster #23("aAO"=w3804) -> (w3799:T10)
                                }
                                n1302 = call "2pparameters.vi"("Params in"=w3799, "command"="set") -> ()  [unwired: 1 out]
                                }
                                frame #1 {
                                n1303 = call "configuration.vi"("command"="get") -> ("config out"=w3809:T11)  [unwired: 2 in, 1 out]
                                n1304 = Unbundle By Name(w3809) -> ("Voltage to Ygalvo"=w3808:i32)
                                n1305 = call "2pparameters.vi"("command"="get") -> ("params out"=w3813:T10)  [unwired: 1 in]
                                n1306 = in-place {
                                in-place-border: w3808 -> [w3818]
                                in-place-border: [w3815] -> w3807
                                n1307 = in-place-cluster #24(w3813) -> ("aAO"=w3817:u32[])
                                n1308 = call "add channel to active arrayv2.vi"("line array in"=w3817, "line to add"=w3818) -> ("line array out"=w3816:u32[], "addition"=w3815:bool)  [unwired: 1 out]
                                n1309 = in-place-cluster #24("aAO"=w3816) -> (w3811:T10)
                                }
                                n1310 = call "2pparameters.vi"("Params in"=w3811, "command"="set") -> ()  [unwired: 1 out]
                                }
                                frame #2 {
                                n1311 = call "2pparameters.vi"("command"="get") -> ("params out"=w3824:T10)  [unwired: 1 in]
